vi "Parse XML Line for Specific Elements.vi"(8 "error in (no error)":errorcluster, 10 "Elements":string[](array[string]), 11 "XML Refnum in":refnum<file>) -> (0 "error out":errorcluster, 1 "Value":string, 2 "Element Name":string, 3 "XML Refnum out":refnum<file>, 4 "Element Found":bool)   [LabVIEW 2013, in "XML Parser.lvclass"]
uses:
  XML Parser.lvclass
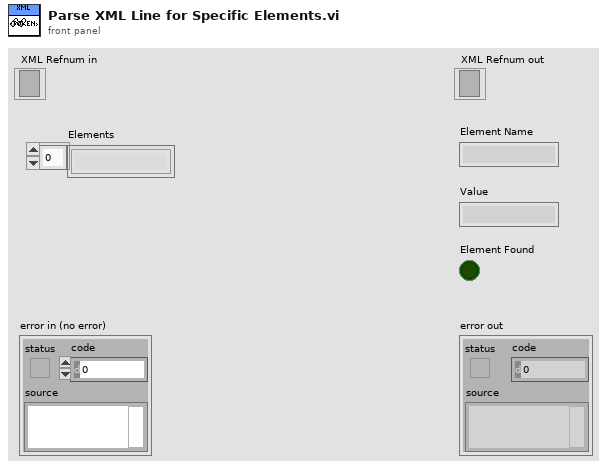
[diagram p1: front panel]
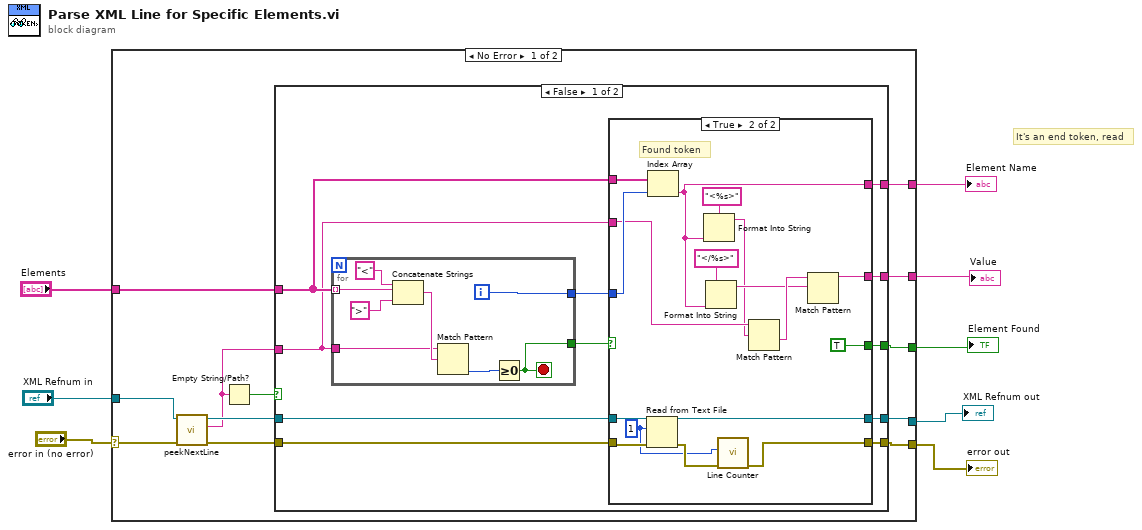
[diagram p0: block diagram]
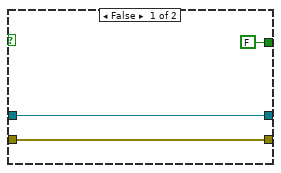
[diagram p2: hidden frame]
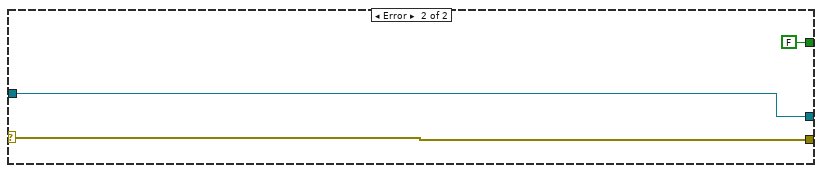
[diagram p4: hidden frame]
diagram:
  # "It's an end token, read"
  n1 = case shown="No Error" "error in (no error)" {
    selector: "error in (no error)" -> [w12 w63]
    tunnel: "XML Refnum in" -> [w13 w64]
    tunnel: "Elements" -> [w18 _]
    tunnel: [w20 w64] -> w5
    tunnel: [w19 w63] -> w2
    tunnel: [w17 _] -> w4
    tunnel: [w16 _] -> w3
    tunnel: [w15 FALSE] -> w1
    frame No Error {
      n2 = call "peekNextLine.vi"("error in"=w12, "file* in"=w13) -> ("error out"=w9:errorcluster, "nextLine"=w11:string, "file* out"=w14:refnum<file>)  [unwired: 7 in]
      n3 = Empty String/Path?(string/path=w11) -> (empty?=w10:bool)
      n4 = case shown="False" w10 {
        tunnel: [w30 w61] -> w20
        tunnel: [w29 w60] -> w19
        tunnel: w18 -> [w28 _]
        tunnel: [w26 _] -> w17
        tunnel: [w25 _] -> w16
        tunnel: [w24 _] -> w15
        tunnel: w14 -> [w23 w61]
        tunnel: w9 -> [w22 w60]
        tunnel: w11 -> [w21 _]
        frame False {
          n5 = for {
            tunnel: w28 -> [w56] mode=indexing
            tunnel: w21 -> [w55]
            tunnel: [w54] -> w31
            tunnel: [w52] -> w27
            i -> [w52]
            stop <- w54 stop-if-true
            n6 = Concatenate Strings("<", w56, ">" ("string")) -> (w59:string)
            n7 = Match Pattern(string=w55, regular expression=w59) -> (offset past match=w53:i32)  [unwired: 1 in, 3 out]
            n8 = Greater Or Equal To 0?(x=w53) -> (x >= 0?=w54:bool)
          }
          n9 = case shown="True" w31 {
            tunnel: w23 -> [w32 w40]
            tunnel: w22 -> [w33 w39]
            tunnel: [w32 w38] -> w30
            tunnel: [w33 w36] -> w29
            tunnel: w28 -> [_ w51]
            tunnel: w27 -> [_ w50]
            tunnel: w21 -> [_ w42]
            tunnel: [_ w45] -> w26
            tunnel: [_ w44] -> w25
            tunnel: [FALSE TRUE] -> w24
            frame False {
            }
            frame True {
              w35 = 1 ("count")
              # "Found token"
              n10 = Read from Text File(file (use dialog)=w40, count=w35, error in=w39) -> (refnum out=w38:refnum<file>, error out=w37:errorcluster)  [unwired: 1 in, 2 out]
              n11 = Index Array(array=w51, index=w50) -> (element=w45:string)
              n12 = Format Into String(format string="<%s>", w45) -> (resulting string=w41:string)  [unwired: 2 in, 1 out]
              n13 = Format Into String(format string="</%s>", w45) -> (resulting string=w46:string)  [unwired: 2 in, 1 out]
              n14 = call "Line Counter.vi"("error in (no error)"=w37, "# of lines to increment (1)"=w35) -> ("error out"=w36:errorcluster)  [unwired: 8 in, 1 out]
              n15 = Match Pattern(string=w42, regular expression=w41) -> (after substring=w47:string)  [unwired: 1 in, 3 out]
              n16 = Match Pattern(string=w47, regular expression=w46) -> (before substring=w44:string)  [unwired: 1 in, 3 out]
            }
          }
        }
        frame True {
        }
      }
    }
    frame Error {
    }
  }
  "XML Refnum out" <- w5
  "error out" <- w2
  "Element Name" <- w4
  "Value" <- w3
  "Element Found" <- w1
